vi "Get DLL path.vi"(8 "error in (no error)":errorcluster, 11 "Skeleton in":refnum<class "Skeleton.lvclass">) -> (0 "error out":errorcluster, 2 "Path":path, 3 "Skeleton out":refnum<class "Skeleton.lvclass">)   [LabVIEW 2016, in "Skeleton.lvlib" / "Skeleton.lvclass"]
uses:
  Skeleton.lvclass
  Skeleton.lvclass/Skeleton.ctl
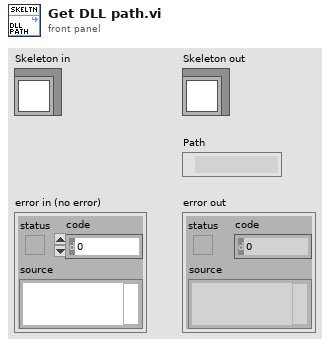
[diagram p1: front panel]
types:
  T1 = typedef "Skeleton.lvlib/Skeleton.lvclass/Private Data.ctl" = cluster{"DLL path":path}
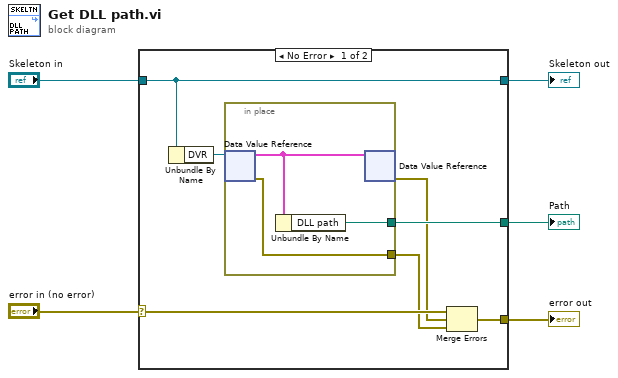
[diagram p0: block diagram]
diagram:
  n1 = case shown="No Error" "error in (no error)" {
    selector: "error in (no error)" -> [w10 w17]
    tunnel: "Skeleton in" -> [w6 w16]
    tunnel: [w12 _] -> w4
    tunnel: [w9 w17] -> w2
    tunnel: [w6 w16] -> w1
    frame No Error {
      n2 = Unbundle By Name(w6) -> ("DVR"=w11:refnum<data-value>)
      n3 = in-place {
        in-place-border: [w14] -> w12
        in-place-border: [w13] -> w7
        n4 = in-place-dvr #1(w11) -> (w15:T1, w13:errorcluster)
        n5 = Unbundle By Name(w15) -> ("DLL path"=w14:path)
        n6 = in-place-dvr #1(w15) -> (w8:errorcluster)  [unwired: 1 out]
      }
      n7 = Merge Errors(w10, w8, w7) -> (w9:errorcluster)
    }
    frame Error {
    }
  }
  "error out" <- w2
  "Skeleton out" <- w1
  "Path" <- w4
